vi "ConfigDlg.vi"(8 "error in (no error)":errorcluster, 11 "FgenPluginsBase in":refnum<class "FgenPluginsBase.lvclass">) -> (0 "error out":errorcluster, 2 "Changed":bool, 3 "FgenPluginsBase out":refnum<class "FgenPluginsBase.lvclass">)   [LabVIEW 2018, in "FgenPlugins.lvlib" / "FgenPluginsBase.lvclass"]
uses:
  FgenPluginsBase.lvclass
panel:
  in  "btnDone":bool
  # "No configurable Parameters for this FGen plugin"
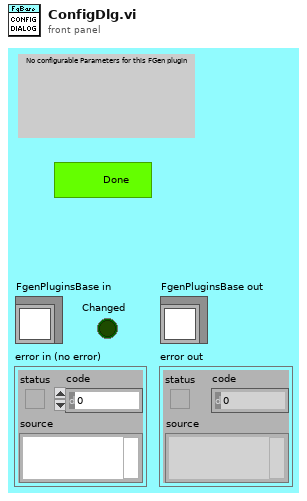
[diagram p1: front panel]
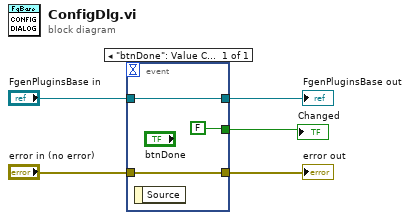
[diagram p0: block diagram]
diagram:
  n1 = event shown="[0] \"btnDone\": Value Change" {
    selector: _ -> [_]
    dyn-events: _ -> [_]
    timeout: _ -> [_]
    tunnel: [FALSE] -> w1
    tunnel: [w7] -> w4
    tunnel: "FgenPluginsBase in" -> [w7]
    tunnel: "error in (no error)" -> [w6]
    tunnel: [w6] -> w2
    event "btnDone": Value Change {
      n2 = event-data() -> ()  [unwired: 1 in, 1 out]
    }
  }
  "error out" <- w2
  "FgenPluginsBase out" <- w4
  "Changed" <- w1
